vi "EditorUndoRedoAction.vi"(7 "Size Ref":refnum<vi>, 8 "error in (no error)":errorcluster, 9 "Undo/Redo":enum16{"Undo", "Redo"}(ring), 10 "UndoRedoCluster":T1, 11 "Board Ref":refnum<vi>) -> (0 "error out":errorcluster)   [LabVIEW 2020]
doc: "Part of Editor.vi\nHandles reaction to undo redo buttons being pressed.\nPasses data between queues, enables/disables buttons as needed and modifies Front Panel acording to data packet from a queue.\nDirection controlled by Undo/Redo Enum input"
uses:
  TypeDef/display-trunct.ctl
  TypeDef/tiles-trunct.ctl
  TypeDef/EditorUndoRedoCluster.ctl
  MessageQueue/QueueRef.ctl
  TypeDef/editor-resize-payload.ctl
  TypeDef/editor-replace-payload.ctl
  <vilib>/Utility/error.llb/Error Cluster From Error Code.vi
  <vilib>/ErrorRing/Error Ring.xnode
  MessageQueue/MessageQueue.lvlib
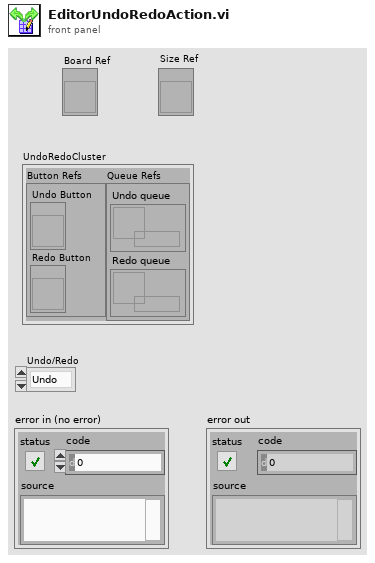
[diagram p1: front panel]
types:
  T1 = typedef "EditorUndoRedoCluster.ctl" = cluster{"Button Refs":cluster{"Undo Button":refnum<vi>, "Redo Button":refnum<vi>}, "Queue Refs":cluster{"Undo queue":T2, "Redo queue":T2}}
  T2 = typedef "MessageQueue.lvlib/QueueRef.ctl" = refnum<queue>
  T3 = enum8{"Enabled", "Disabled", "Disabled and Grayed Out"}
  T4 = typedef "editor-resize-payload.ctl" = cluster{"Old Board":T5, "New Board":T5}
  T5 = typedef "display-trunct.ctl" = T6[][]
  T6 = typedef "tiles-trunct.ctl" = u16
  T7 = typedef "editor-replace-payload.ctl" = cluster{"row":i32, "col":i32, "Old Tile":T6, "New Tile":T6}
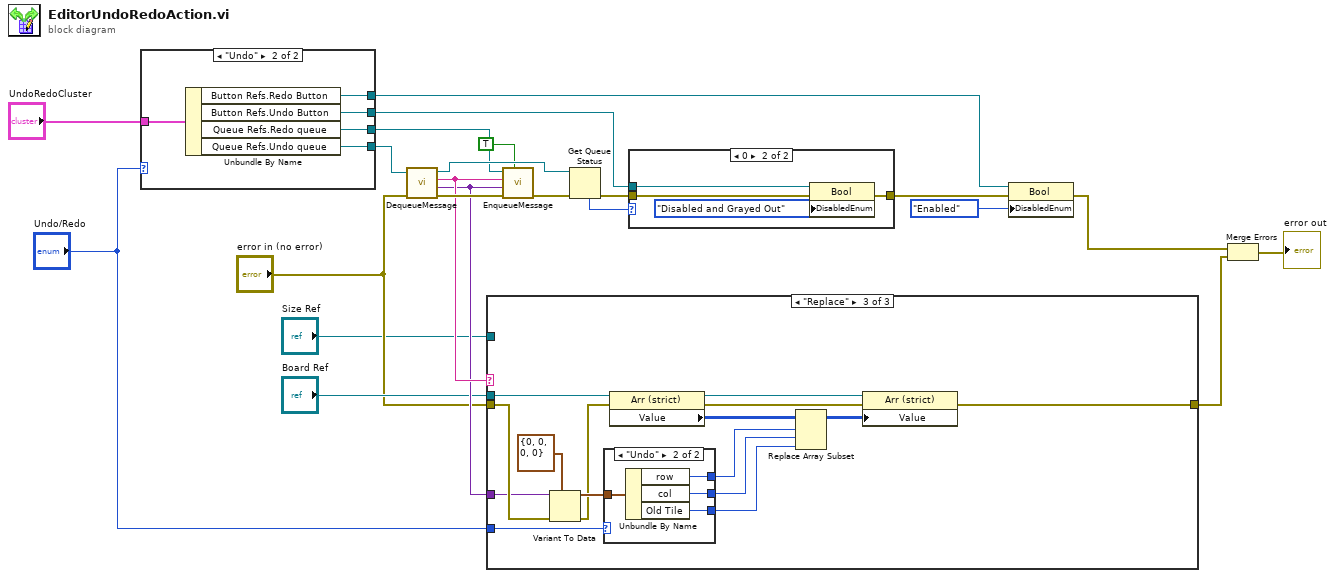
[diagram p0: block diagram]
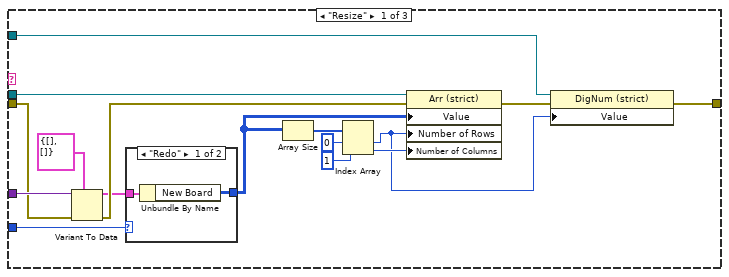
[diagram p2: hidden frame]
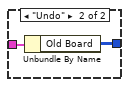
[diagram p3: hidden frame]
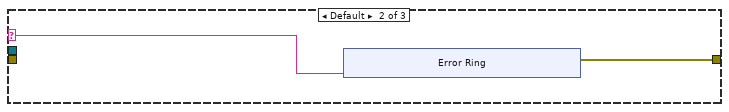
[diagram p4: hidden frame]
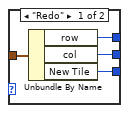
[diagram p5: hidden frame]
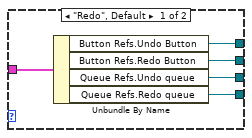
[diagram p6: hidden frame]
diagram:
  n1 = case shown="\"Undo\"" "Undo/Redo" {
    tunnel: "UndoRedoCluster" -> [w27 w32]
    tunnel: [w26 w31] -> w13
    tunnel: [w25 w30] -> w12
    tunnel: [w24 w28] -> w10
    tunnel: [w23 w29] -> w11
    frame "Redo", Default {
      n2 = Unbundle By Name(w27) -> ("Button Refs.Undo Button"=w23:refnum<vi>, "Button Refs.Redo Button"=w24:refnum<vi>, "Queue Refs.Undo queue"=w26:T2, "Queue Refs.Redo queue"=w25:T2)
    }
    frame "Undo" {
      n3 = Unbundle By Name(w32) -> ("Button Refs.Redo Button"=w29:refnum<vi>, "Button Refs.Undo Button"=w28:refnum<vi>, "Queue Refs.Redo queue"=w31:T2, "Queue Refs.Undo queue"=w30:T2)
    }
  }
  n4 = call "DequeueMessage.vi"("error in (no error)"="error in (no error)", "queue in"=w12) -> ("error out"=w17:errorcluster, "Data (Variant)"=w8:variant, "Message"=w9:string, "queue out (copy)"=w19:T2)  [unwired: 6 in]
  n5 = case shown="\"Replace\"" w9 {
    selector: w9 -> [_ w53 _]
    tunnel: w8 -> [w47 _ w69]
    tunnel: "Board Ref" -> [w48 _ w76]
    tunnel: "error in (no error)" -> [w45 _ w70]
    tunnel: [w35 w54 w74] -> w5
    tunnel: "Undo/Redo" -> [w42 _ w68]
    tunnel: "Size Ref" -> [w34 _ _]
    frame "Resize" {
      n6 = Variant To Data(error in=w45, type=T4 {"Old Board"=[], "New Board"=[]} ("Resize Payload"), Variant=w47) -> (data=w43:T4, error out=w44:errorcluster)
      n7 = case shown="\"Redo\"" w42 {
        tunnel: w43 -> [w50 w52]
        tunnel: [w49 w51] -> w41
        frame "Redo" {
          n8 = Unbundle By Name(w50) -> ("New Board"=w49:T5)
        }
        frame "Undo" {
          n9 = Unbundle By Name(w52) -> ("Old Board"=w51:T5)
        }
      }
      n10 = Array Size(array=w41) -> (size(s)=w40:i32[])
      n11 = Index Array(array=w40, index #1=0 ("index"), index #2=1 ("index")) -> (element #1=w33:i32, element #2=w37:i32)
      n12 = property class="Arr (strict)"(reference=w48, error in=w44, "Value"=w41, "Number of Rows"=w33, "Number of Columns"=w37) -> (error out=w36:errorcluster)  [unwired: 1 out]
      n13 = property class="DigNum (strict)"(reference=w34, error in=w36, "Value"=w33) -> (error out=w35:errorcluster)  [unwired: 1 out]
    }
    frame Default {
      n14 = xnode "Error Ring"("parameter 0"=w53) -> ("error out"=w54:errorcluster)
    }
    frame "Replace" {
      n15 = Variant To Data(error in=w70, type=T7 {"row"=0, "col"=0, "Old Tile"=0, "New Tile"=0} ("Replace Payload"), Variant=w69) -> (data=w72:T7, error out=w67:errorcluster)
      n16 = case shown="\"Undo\"" w68 {
        tunnel: w72 -> [w80 w84]
        tunnel: [w79 w83] -> w65
        tunnel: [w78 w82] -> w64
        tunnel: [w77 w81] -> w63
        frame "Redo" {
          n17 = Unbundle By Name(w80) -> ("row"=w79:i32, "col"=w78:i32, "New Tile"=w77:T6)
        }
        frame "Undo" {
          n18 = Unbundle By Name(w84) -> ("row"=w83:i32, "col"=w82:i32, "Old Tile"=w81:T6)
        }
      }
      n19 = property class="Arr (strict)"(reference=w76, error in=w67) -> (reference out=w75:refnum<vi>, error out=w62:errorcluster, "Value"=w73:T5)
      n20 = Replace Array Subset(array=w73, new element=w63, index (row)=w65, index (col)=w64) -> (w66:T5)
      n21 = property class="Arr (strict)"(reference=w75, error in=w62, "Value"=w66) -> (error out=w74:errorcluster)  [unwired: 1 out]
    }
  }
  n22 = call "EnqueueMessage.vi"("Priority? (F)"=TRUE, "error in (no error)"=w17, "Data"=w8, "Message"=w9, "queue in"=w13) -> ("error out"=w18:errorcluster)  [unwired: 5 in, 1 out]
  n23 = Get Queue Status(queue=w19, error in (no error)=w18) -> (error out=w22:errorcluster, # elements in queue=w20:i32)  [unwired: 1 in, 6 out]
  n24 = case shown="0" w20 {
    tunnel: [w85 w89] -> w21
    tunnel: w22 -> [w85 w88]
    tunnel: w10 -> [_ w86]
    frame Default {
    }
    frame 0 {
      n25 = property on="Property Node" class="Bool"(reference=w86, error in=w88, "DisabledEnum"=T3."Disabled and Grayed Out" ("Disabled")) -> (error out=w89:errorcluster)  [unwired: 1 out]
    }
  }
  n26 = property on="Property Node" class="Bool"(reference=w11, error in=w21, "DisabledEnum"=T3."Enabled" ("Disabled")) -> (error out=w15:errorcluster)  [unwired: 1 out]
  n27 = Merge Errors(w15, w5) -> (→"error out":errorcluster)
